vi "CV07_generator.vi"() -> (1 "Original Sine 60 Hz":waveform(dbl), 3 "Signal for filtration":waveform(dbl))   [LabVIEW 2023]
uses:
  <vilib>/measure/NI_MABase.lvlib
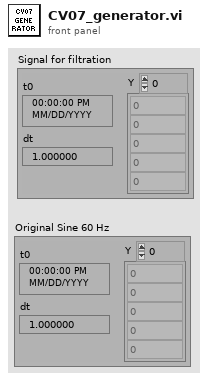
[diagram p1: front panel]
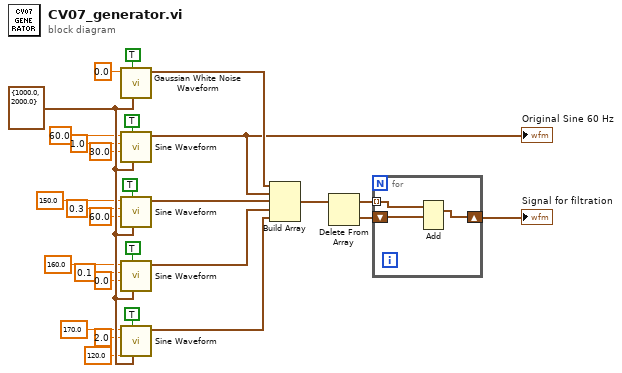
[diagram p0: block diagram]
diagram:
  w28 = cluster{"Fs":dbl, "#s":dbl} {"Fs"=1000.0, "#s"=2000.0} ("sampling info")
  n1 = call <vilib>:"Gaussian White Noise Waveform.vi"("sampling info"=w28, "reset signal"=TRUE, "standard deviation"=0.0) -> ("signal out"=w2:waveform(dbl))  [unwired: 7 in, 1 out]
  n2 = call <vilib>:"Sine Waveform.vi"("sampling info"=w28, "reset signal"=TRUE, "phase"=30.0, "amplitude"=1.0, "frequency"=60.0) -> ("signal out"=w1:waveform(dbl))  [unwired: 5 in, 1 out]
  "Original Sine 60 Hz" <- w1
  n3 = call <vilib>:"Sine Waveform.vi"("sampling info"=w28, "reset signal"=TRUE, "phase"=60.0, "amplitude"=0.3, "frequency"=150.0) -> ("signal out"=w7:waveform(dbl))  [unwired: 5 in, 1 out]
  n4 = call <vilib>:"Sine Waveform.vi"("sampling info"=w28, "reset signal"=TRUE, "phase"=0.0, "amplitude"=0.1, "frequency"=160.0) -> ("signal out"=w8:waveform(dbl))  [unwired: 5 in, 1 out]
  n5 = call <vilib>:"Sine Waveform.vi"("sampling info"=w28, "reset signal"=TRUE, "phase"=120.0, "amplitude"=2.0, "frequency"=170.0) -> ("signal out"=w9:waveform(dbl))  [unwired: 5 in, 1 out]
  n6 = Build Array(w2, w1, w7, w8, w9) -> (w6:waveform(dbl)[])
  n7 = Delete From Array(array=w6) -> (deleted portion=w5:waveform(dbl), array with subset deleted=w4:waveform(dbl)[])  [unwired: 2 in]
  n8 = for {
    tunnel: w4 -> [w30] mode=indexing
    shift-right: [w29] -> w3
    shift-left: w5 -> [w31]
    n9 = Add(1:w31, 2:w30) -> (0:w29:waveform(dbl))  [unwired: 1 in, 1 out]
  }
  "Signal for filtration" <- w3
